vi "Waveform Flatten.vi"(7 "payload in":u8[](array[numeric]), 8 "error in (no error)":errorcluster, 9 "FIFO Timestamps":T1, 10 "Data in":T2[](array[typedef]), 11 "CIFChannels in":refnum<class "CIFChannels.lvclass">) -> (0 "error out":errorcluster, 1 "Total Length":i32, 2 "Data out":T2[](array[typedef]), 3 "CIFChannels out":refnum<class "CIFChannels.lvclass">, 5 "payload out":u8[](array[numeric]))   [LabVIEW 2021]
uses:
  typedef/Datatype Waveform.ctl
  typedef/TimeStamps.ctl
  CIFChannels/CIFChannels.lvclass
  CIFChannels/CIFChannels.lvclass/CIFChannels.ctl
  be24e584-1bb9-4ddb-b1ad-5fa4498d0a1e.vi
  be24e584-1bb9-4ddb-b1ad-5fa4498d0a1e.vi/c28b0ead-42ad-4072-80a2-aca7f2bd7ce3.vi
  Utilities/Flatten Header.vi
  CIFChannels/Utilities/Update FIFO Header.vi
  <vilib>/CIF Foundation/CIF Utilities/Time/System Time/Get System Time.vi
  <vilib>/CIF Foundation/CIF Utilities/Time/System Time/LabVIEW Time to TAI Time.vi
  <vilib>/CIF Foundation/CIF Utilities/DataTypes/DataTypes_CIF_U.lvlib
  ChannelCommon.lvlib
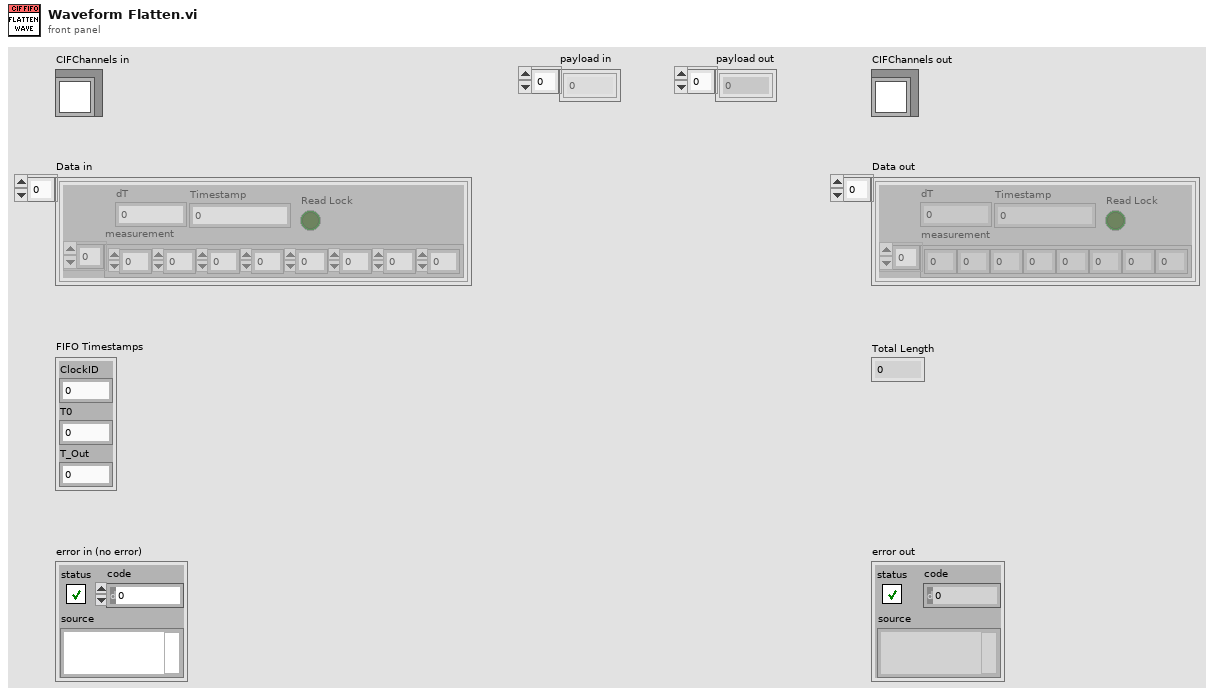
[diagram p1: front panel]
types:
  T1 = typedef "ChannelCommon.lvlib/TimeStamps.ctl" = cluster{"ClockID":u8, "T0":i64, "T_Out":i64}
  T2 = typedef "ChannelCommon.lvlib/Datatype Waveform.ctl" = cluster{"measurement":dbl[], "dT":dbl, "Timestamp":i64, "Read Lock":bool}
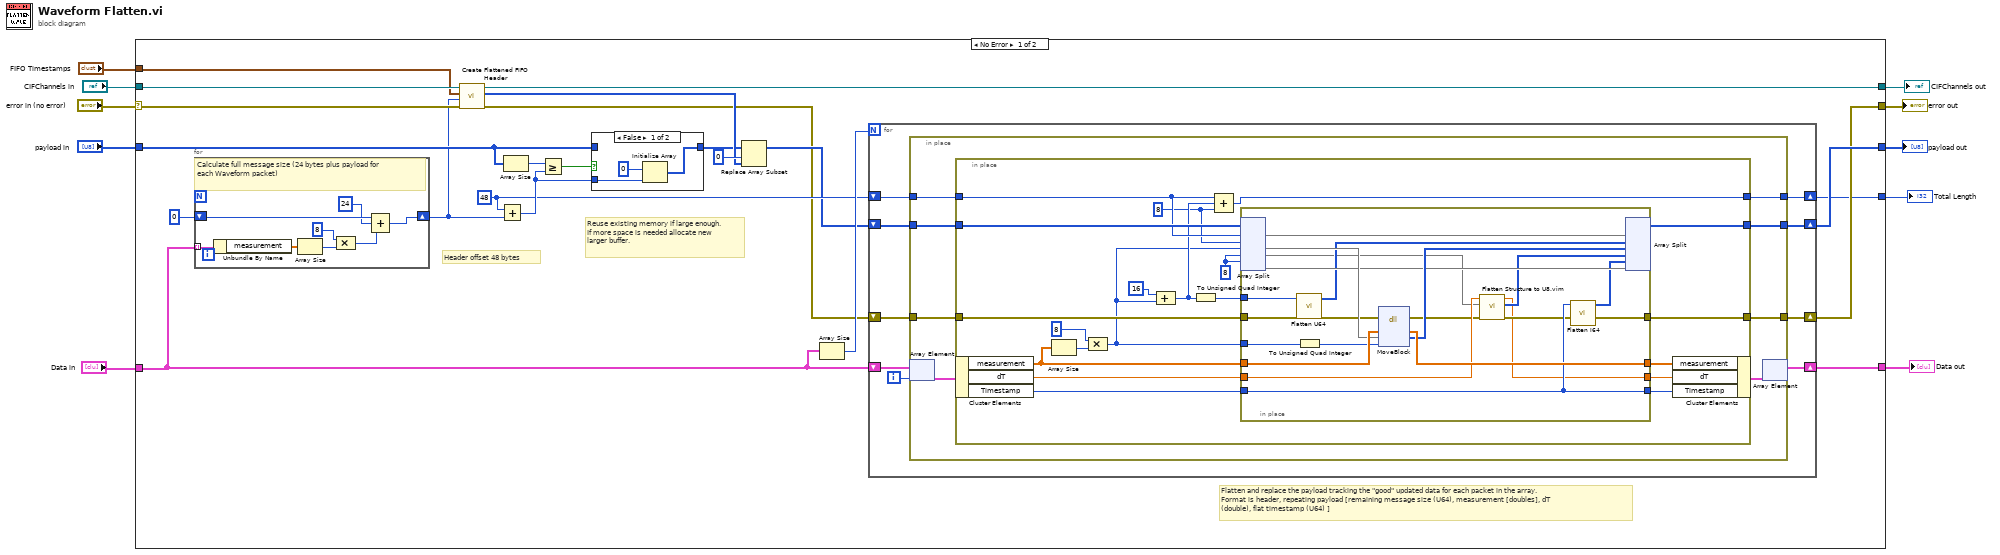
[diagram p0: block diagram]
diagram:
  n1 = case shown="No Error" "error in (no error)" {
    selector: "error in (no error)" -> [w19 w104]
    tunnel: [w26 w104] -> w9
    tunnel: "Data in" -> [w21 w101]
    tunnel: "CIFChannels in" -> [w20 w103]
    tunnel: [w16 w103] -> w2
    tunnel: [w27 w102] -> w8
    tunnel: "payload in" -> [w29 w102]
    tunnel: [w25 w101] -> w5
    tunnel: [w23 _] -> w4
    tunnel: "FIFO Timestamps" -> [w11 _]
    frame No Error {
      w24 = 48 ("y")
      # "Flatten and replace the payload tracking the \"good\" updated data for each packet in the array.\nFormat is header, repeating payload [remaining message size (U64), measurement [doubles], dT (double), flat timestamp (U64) ]"
      # "Header offset 48 bytes"
      # "Reuse existing memory if large enough.  If more space is needed allocate new larger buffer."
      n2 = for {
        tunnel: w21 -> [w40] mode=indexing
        shift-right: [w38] -> w18
        shift-left: 0 -> [w37]
        # "Calculate full message size (24 bytes plus payload for each Waveform packet)"
        n3 = Unbundle By Name(w40) -> ("measurement"=w39:dbl[])
        n4 = Array Size(array=w39) -> (size(s)=w35:i32)
        n5 = Compound Arithmetic op=MULTIPLY(8 ("value"), w35) -> (w34:i32)
        n6 = Compound Arithmetic op=ADD(w37, 24 ("value"), w34) -> (w38:i32)
      }
      n7 = call "Create Flattened FIFO Header.vi"("error in (no error)"=w19, "Data Length"=w18, "FIFO Timestamps"=w11, "CIFChannels in"=w20) -> ("error out"=w12:errorcluster, "Flattened FIFO Header"=w15:u8[], "CIFChannels out"=w16:refnum<class "CIFChannels.lvclass">)  [unwired: 5 in]
      n8 = Add(x=w24, y=w18) -> (x+y=w30:i32)
      n9 = Array Size(array=w29) -> (size(s)=w32:i32)
      n10 = Greater Or Equal?(x=w32, y=w30) -> (x >= y?=w31:bool)
      n11 = case shown="False" w31 {
        tunnel: w29 -> [_ w100]
        tunnel: [w97 w100] -> w14
        tunnel: w30 -> [w99 _]
        frame False {
          n12 = Initialize Array(u8 0, w99) -> (w97:u8[])
        }
        frame True {
        }
      }
      n13 = Replace Array Subset(array=w14, new element=w15, index=0) -> (w13:u8[])
      n14 = Array Size(array=w21) -> (size(s)=w28:i32)
      n15 = for {
        N: w28 -> [_]
        shift-right: [w49] -> w26
        shift-left: w12 -> [w48]
        shift-right: [w46] -> w27
        shift-left: w13 -> [w47]
        shift-right: [w44] -> w23
        shift-left: w24 -> [w45]
        shift-right: [w41] -> w25
        shift-left: w21 -> [w43]
        i -> [w42]
        n16 = in-place {
          in-place-border: [w57] -> w49
          in-place-border: w48 -> [w56]
          in-place-border: w47 -> [w55]
          in-place-border: [w54] -> w46
          in-place-border: w45 -> [w53]
          in-place-border: [w52] -> w44
          n17 = in-place-array #1(w43, w42) -> (w51:T2)
          n18 = in-place {
            in-place-border: [w77] -> w57
            in-place-border: w56 -> [w76]
            in-place-border: w55 -> [w75]
            in-place-border: [w74] -> w54
            in-place-border: w53 -> [w73]
            in-place-border: [w72] -> w52
            w58 = 8
            w60 = 8
            n19 = in-place-cluster #2(w51) -> ("measurement"=w69:dbl[], "dT"=w68:dbl, "Timestamp"=w67:i64)
            n20 = Array Size(array=w69) -> (size(s)=w62:i32)
            n21 = Compound Arithmetic op=MULTIPLY(8 ("value"), w62) -> (w61:i32)
            n22 = Compound Arithmetic op=ADD(16 ("value"), w61) -> (w70:i32)
            n23 = To Unsigned Quad Integer(1:w70) -> (0:w59:u64)
            n24 = Compound Arithmetic op=ADD(w73, w70, w58) -> (w72:i32)
            n25 = in-place {
              in-place-border: w67 -> [w84]
              in-place-border: w76 -> [w86]
              in-place-border: [w80] -> w77
              in-place-border: w69 -> [w95]
              in-place-border: w68 -> [w83]
              in-place-border: w59 -> [w88]
              in-place-border: [w94] -> w66
              in-place-border: [w78] -> w65
              in-place-border: [w84] -> w64
              in-place-border: w61 -> [w93]
              n26 = in-place-split #3(w75, w73, w58, w61, w60, w60) -> (w96:u8[], w91:u8[], w82:u8[], w89:u8[])  [unwired: 2 out]
              n27 = call <vilib>:"Flatten U64.vi"("U64"=w88) -> ("Flat Data"=w87:u8[])  [unwired: 4 in]
              n28 = To Unsigned Quad Integer(1:w93) -> (0:w92:u64)
              n29 = dll-call lib="LabVIEW" fn="MoveBlock"(error in=w86, "source"=w95, "dest"=w91, "size"=w92) -> (error out=w81:errorcluster, "source"=w94:dbl[], "dest"=w90:u8[])  [unwired: 4 in, 1 out]
              n30 = call "Flatten Structure to U8.vim"("error in"=w81, "Flattened Data in"=w82, "Data to Flatten in"=w83) -> ("error out"=w80:errorcluster, "Flattened Data out"=w79:u8[], "Data to Flatten out"=w78:dbl)  [unwired: 6 in]
              n31 = call <vilib>:"Flatten I64.vi"("I64"=w84) -> ("Flat Data"=w85:u8[])  [unwired: 4 in]
              n32 = in-place-split #3(w96, w87, w90, w79, w85, w89) -> (w74:u8[])  [unwired: 5 out]
            }
            n33 = in-place-cluster #2("measurement"=w66, "dT"=w65, "Timestamp"=w64) -> (w50:T2)
          }
          n34 = in-place-array #1(w50) -> (w41:T2[])  [unwired: 1 out]
        }
      }
    }
    frame Error {
    }
  }
  "error out" <- w9
  "payload out" <- w8
  "Data out" <- w5
  "Total Length" <- w4
  "CIFChannels out" <- w2
